vi "copyright.vi"(2 "year":u16) -> ()   [LabVIEW 2015]
uses:
  toolbar icons/help.ctl
  <vilib>/Platform/browser.llb/Open URL in Default Browser (string).vi
panel:
  in  "Help Button":T1
  in  "OK Button":bool
  out "Info":string
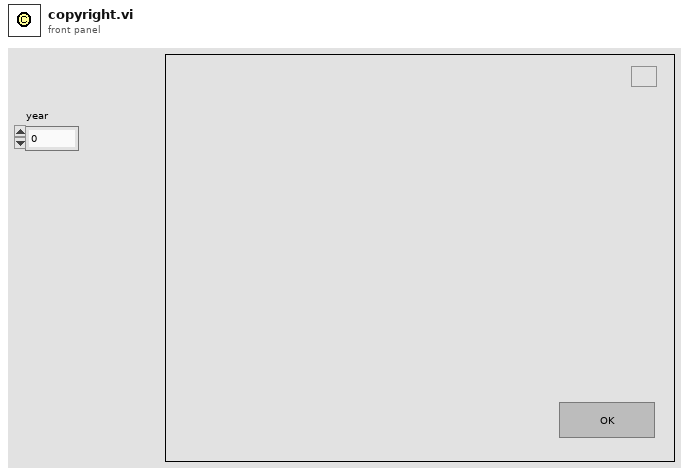
[diagram p1: front panel]
types:
  T1 = typedef "help.ctl" = bool
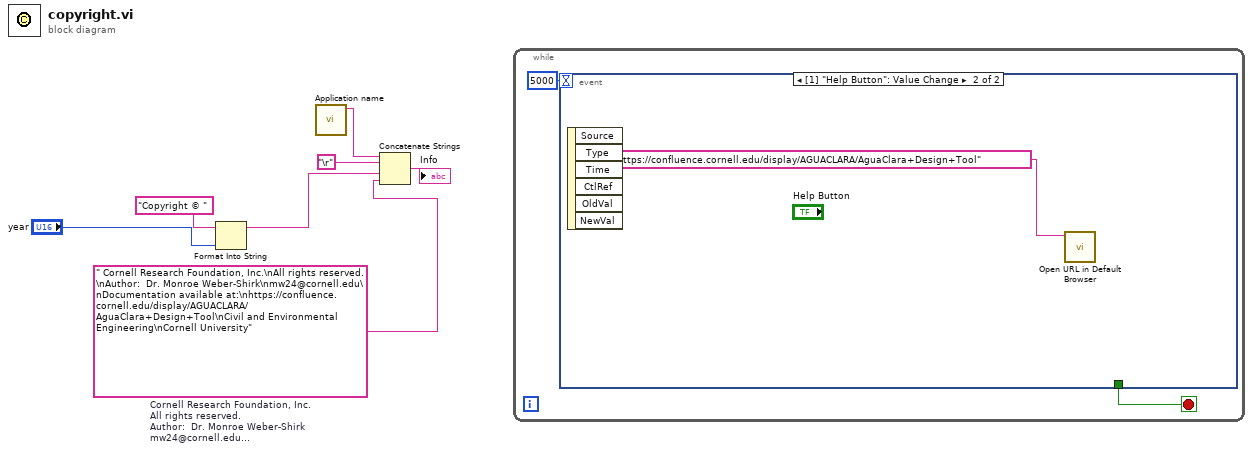
[diagram p0: block diagram]
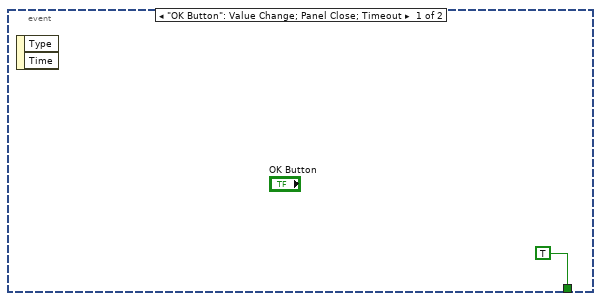
[diagram p2: hidden frame]
diagram:
  w4 = " Cornell Research Foundation, Inc.\nAll rights reserved.\nAuthor:  Dr. Monroe Weber-Shirk\nmw24@cornell.edu\nDocumentation available at:\nhttps://confluence.cornell.edu/display/AGUACLARA/AguaClara+Design+Tool\nCivil and Environmental Engineering\nCornell University"  # Cornell Research Foundation, Inc. All rights reserved. Author:  Dr. Monroe Weber-Shirk mw24@cornell.edu Documentation available at: https://confluence.cornell.edu/display/AGUACLARA/AguaClara+Design+Tool Civil and Environmental Engineering Cornell University
  n1 = Format Into String(initial string="Copyright © ", "year") -> (resulting string=w5:string)  [unwired: 2 in, 1 out]
  n2 = call "Application name.vi"() -> ("application name"=w2:string)  [unwired: 5 in, 2 out]
  n3 = Concatenate Strings(w2, "\r", w5, w4) -> (→"Info":string)
  n4 = while {
    stop <- w9 stop-if-true
    n5 = event shown="[1] \"Help Button\": Value Change" {
      selector: _ -> [_ _]
      dyn-events: _ -> [_ _]
      timeout: 5000 -> [_ _]
      tunnel: [TRUE _] -> w9
      event "OK Button": Value Change; Panel Close; Timeout {
        n6 = event-data() -> ()  [unwired: 1 in, 2 out]
      }
      event Value Change {
        n7 = event-data() -> ()  [unwired: 1 in, 6 out]
        n8 = call-poly <vilib>:"Open URL in Default Browser.vi"("URL"="https://confluence.cornell.edu/display/AGUACLARA/AguaClara+Design+Tool") -> ()  [unwired: 5 in, 2 out]
      }
    }
  }
